vi "DQMH System Message - Ready for Display.vi"(8 "Target SP Name":string="SP_Content", 9 "Title":string="<not specified>", 10 "Main VI Reference":refnum<vi>) -> (1 "Payload":variant, 2 "Identifier":string="Ready for Display", 5 "Source":T1)   [LabVIEW 2022 SP3, in "hse-dqmh.lvlib"]
doc: "____\nHAMPEL SOFTWARE ENGINEERING v3.8.0 (2023-12-18 14:41)"
uses:
  hse-dqmh.lvlib
  Controls/System Message Source.ctl
  Controls/System Message Framework Identifiers.ctl
  Controls/System Message - Ready for Display - Payload--cluster.ctl
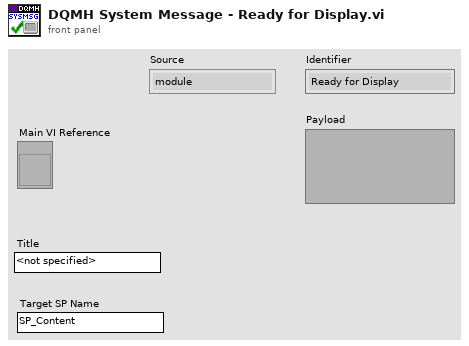
[diagram p1: front panel]
types:
  T1 = typedef "hse-dqmh.lvlib/System Message Source.ctl" = enum16{"module", "application", "network"}
  T2 = typedef "hse-dqmh.lvlib/System Message - Ready for Display - Payload--cluster.ctl" = cluster{"Module Path":path, "VI Reference":refnum<vi>, "Title":string, "Target SP Name":string}
  T3 = typedef "hse-dqmh.lvlib/System Message Framework Identifiers.ctl" = enum16{"Add to Run-Time Menu", "Ready for Display", "Removed from Subpanel", "Remove from Run-Time Menu"}
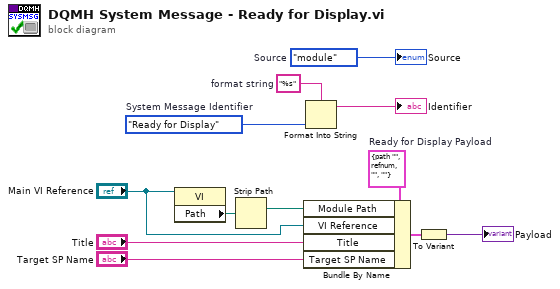
[diagram p0: block diagram]
diagram:
  w7 = T2 {"Module Path"=path "", "VI Reference"=refnum, "Title"="", "Target SP Name"=""}  # Ready for Display Payload
  w10 = "%s"  # format string
  w9 = System_Message_Framework_Identifiers."Ready for Display"  # System Message Identifier
  w12 = System_Message_Source."module"  # Source
  n1 = property class="VI"(reference="Main VI Reference") -> ("Path"=w5:path)  [unwired: 1 in, 2 out]
  n2 = Strip Path(path=w5) -> (stripped path=w4:path)  [unwired: 1 out]
  n3 = Bundle By Name(cluster=w7, "Module Path"=w4, "VI Reference"="Main VI Reference", "Title"="Title", "Target SP Name"="Target SP Name") -> (w6:T2)
  n4 = Format Into String(format string=w10, w9) -> (resulting string=→"Identifier":string)  [unwired: 2 in, 1 out]
  n5 = To Variant(anything=w6) -> (Variant=→"Payload":variant)
  "Source" <- w12
